vi "Title.vi"(8 "error in (no error)":errorcluster, 11 "List Box View Model in":refnum<class "Multicolumn List Box View Model.lvclass">) -> (0 "error out":errorcluster, 2 "Title":string, 3 "List Box View Model out":refnum<class "Multicolumn List Box View Model.lvclass">)   [LabVIEW 2020, in "Multicolumn List Box View Model.lvclass"]
uses:
  Multicolumn List Box View Model.lvclass
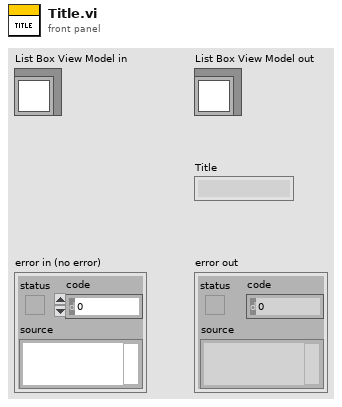
[diagram p1: front panel]
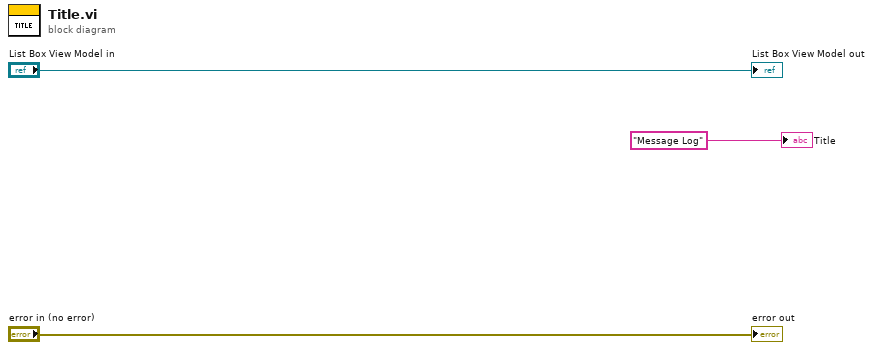
[diagram p0: block diagram]
diagram:
  "error out" <- "error in (no error)"
  "List Box View Model out" <- "List Box View Model in"
  "Title" <- "Message Log"
